vi "CSTK_Enum_Creator.vi"(10 "应用程序:菜单启动:VI":string, 11 "应用程序引用（本地）":refnum<vi>) -> ()   [LabVIEW 2015, in "CSTK_Enum Creator.lvlib"]
uses:
  CSTK_Enum Creator.lvlib
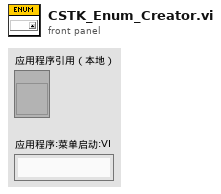
[diagram p1: front panel]
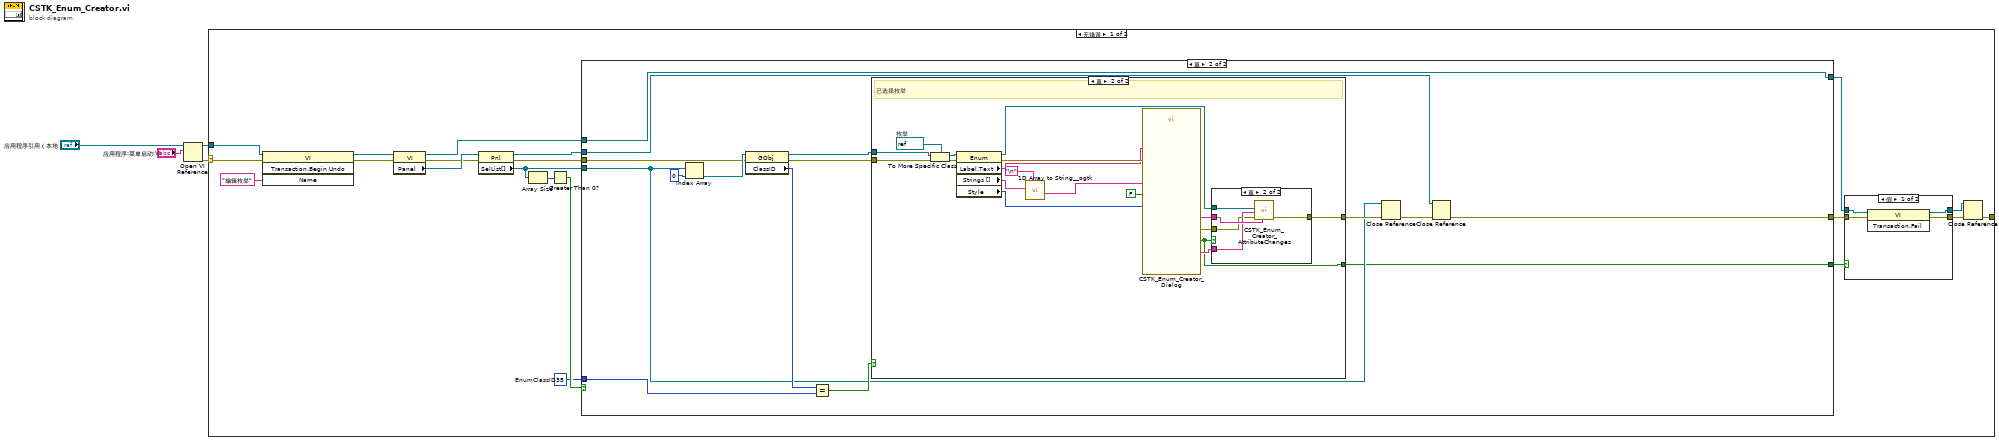
[diagram p0: block diagram]
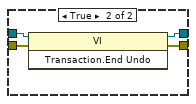
[diagram p2: hidden frame]
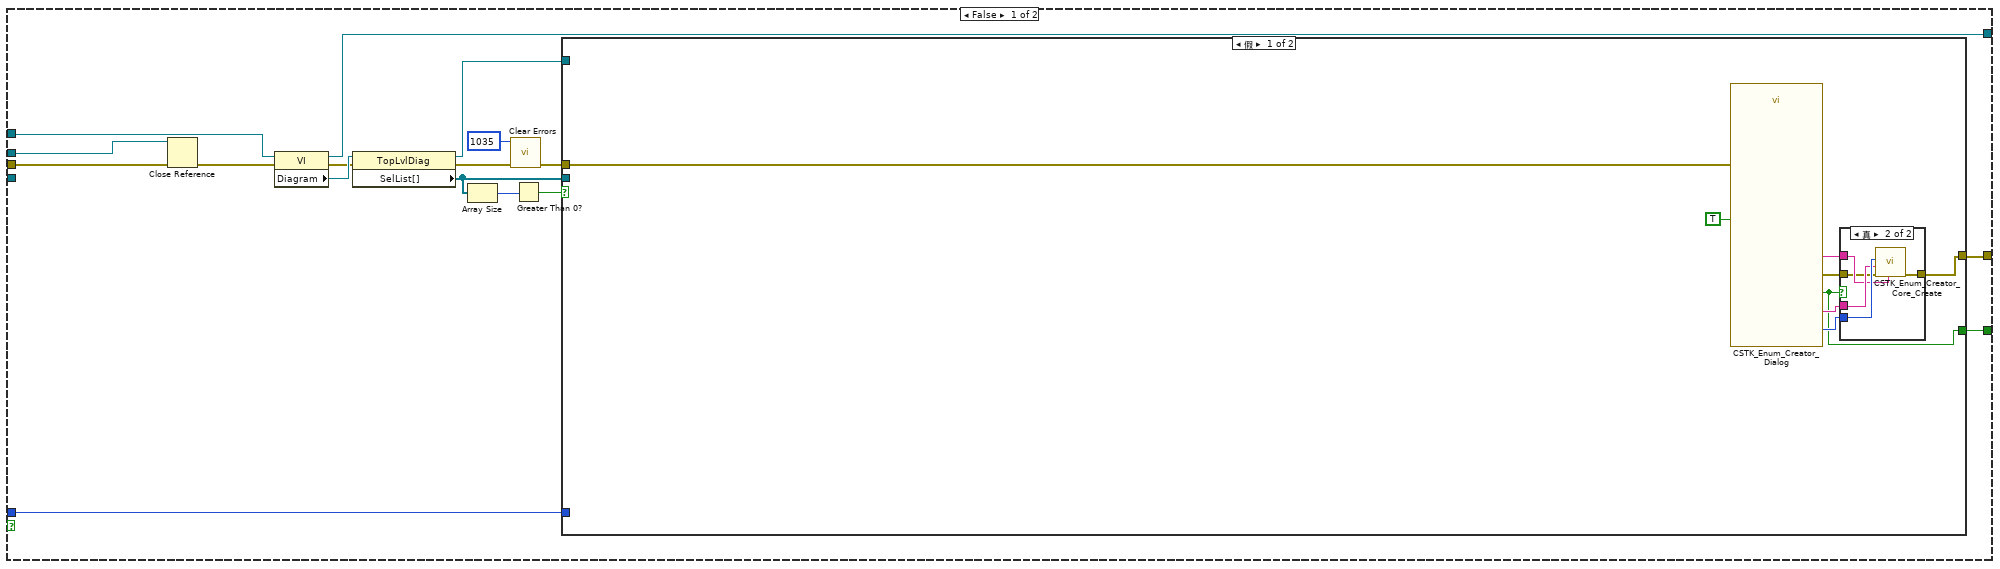
[diagram p3: hidden frame]
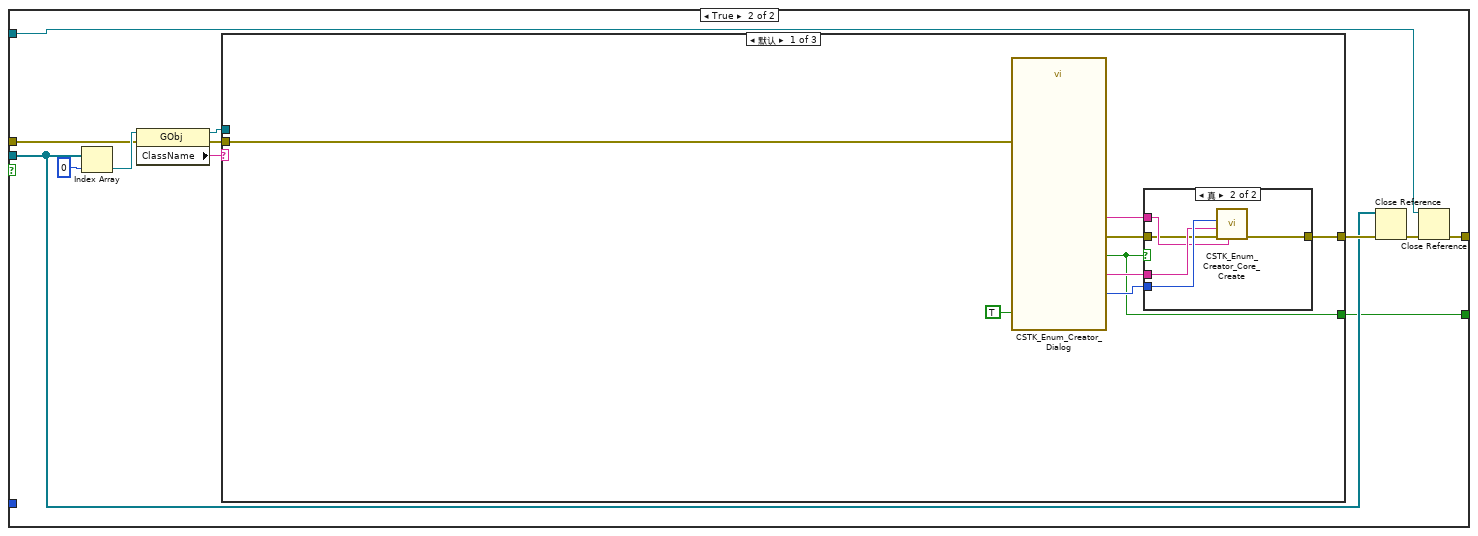
[diagram p5: hidden frame]
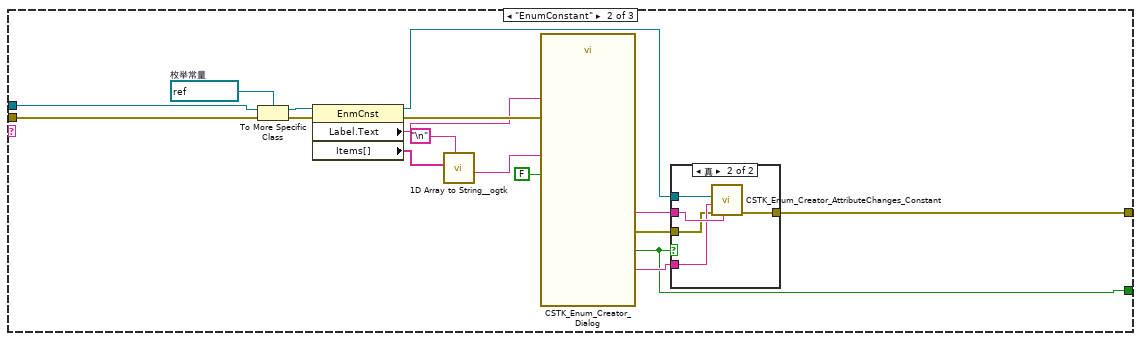
[diagram p7: hidden frame]
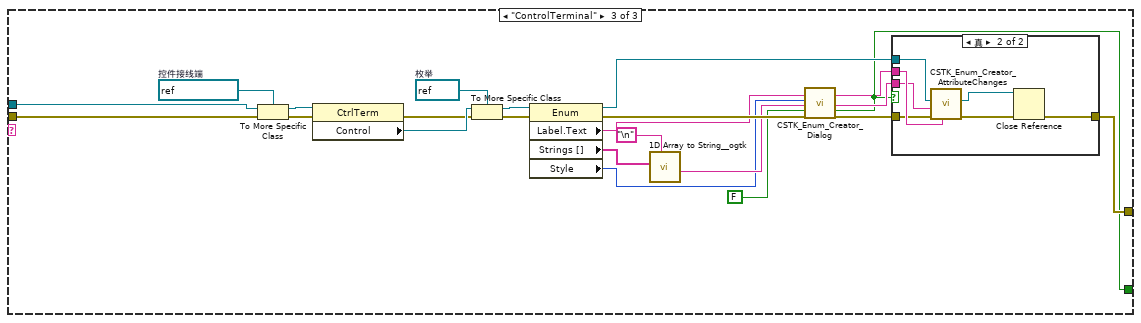
[diagram p9: hidden frame]
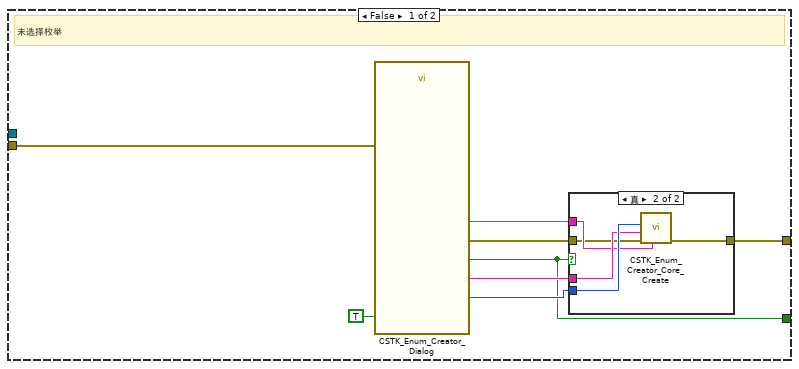
[diagram p11: hidden frame]
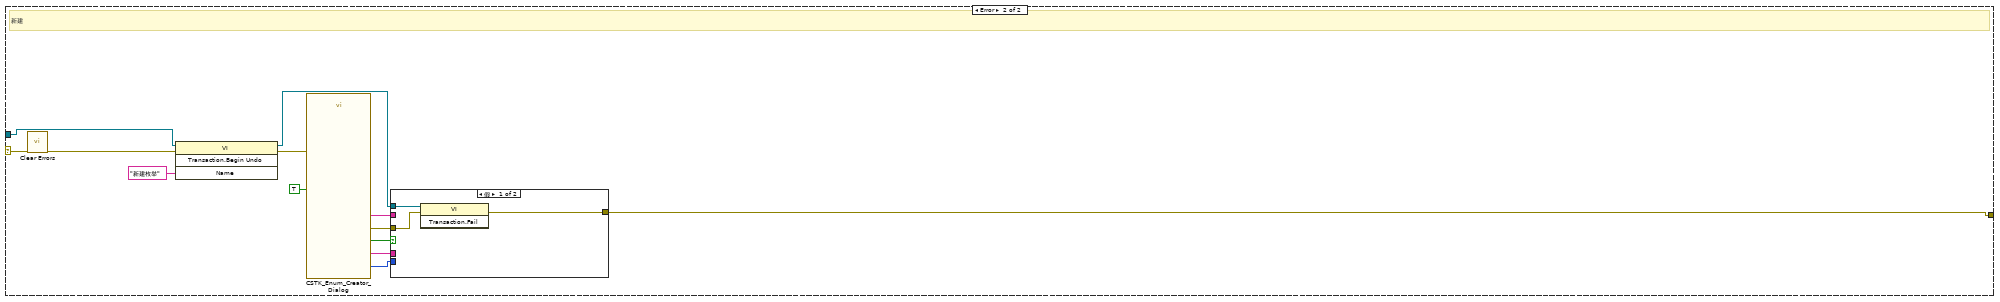
[diagram p14: hidden frame]
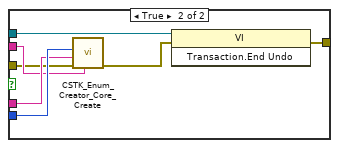
[diagram p15: hidden frame]
diagram:
  n1 = Open VI Reference(application reference (local)="应用程序引用（本地）", vi path="应用程序:菜单启动:VI") -> (vi reference=w1:refnum<vi>, error out=w3:errorcluster)  [unwired: 4 in]
  n2 = case shown="无错误" w3 {
    selector: w3 -> [w13 w209]
    tunnel: w1 -> [w14 w200]
    tunnel: [w21 w202] -> _
    frame No Error {
      w15 = u32 35  # EnumClassID
      n3 = invoke class="VI" method="Transaction.Begin Undo"(reference=w14, error in=w13, "Name"="编辑枚举" ("名称")) -> (reference out=w12:refnum<vi>, error out=w11:errorcluster)  [unwired: 1 in, 2 out]
      n4 = property class="VI"(reference=w12, error in=w11) -> (reference out=w17:refnum<vi>, error out=w22:errorcluster, "Panel"=w24:refnum<vi>)
      n5 = property class="Pnl"(reference=w24, error in=w22) -> (reference out=w16:refnum<vi>, error out=w23:errorcluster, "SelList[]"=w20:refnum<vi>[])
      n6 = Array Size(array=w20) -> (size(s)=w19:i32)
      n7 = Greater Than 0?(x=w19) -> (x > 0?=w18:bool)
      n8 = case shown="真" w18 {
        tunnel: w23 -> [w36 w153]
        tunnel: [w41 w147] -> w7
        tunnel: w20 -> [_ w150]
        tunnel: w17 -> [w49 w149]
        tunnel: [w46 w149] -> w9
        tunnel: w16 -> [w45 w146]
        tunnel: w15 -> [w38 w145]
        tunnel: [w35 w144] -> w5
        frame False {
          n9 = Close Reference(reference=w45, error in (no error)=w36) -> (error out=w44:errorcluster)
          n10 = property class="VI"(reference=w49, error in=w44) -> (reference out=w46:refnum<vi>, error out=w47:errorcluster, "Diagram"=w48:refnum<vi>)
          n11 = property class="TopLvlDiag"(reference=w48, error in=w47) -> (reference out=w37:refnum<vi>, error out=w40:errorcluster, "SelList[]"=w39:refnum<vi>[])
          n12 = Array Size(array=w39) -> (size(s)=w43:i32)
          n13 = call <vilib>:"Clear Errors.vi"("error in (no error)"=w40, "specific error code to clear (0: all)"=1035) -> ("error out"=w34:errorcluster)  [unwired: 4 in, 1 out]
          n14 = Greater Than 0?(x=w43) -> (x > 0?=w42:bool)
          n15 = case shown="假" w42 {
            tunnel: [w51 w73] -> w41
            tunnel: w34 -> [w52 w65]
            tunnel: w39 -> [_ w71]
            tunnel: w38 -> [_ _]
            tunnel: w37 -> [_ w70]
            tunnel: [w50 w64] -> w35
            frame False {
              n16 = call "CSTK_Enum_Creator_Dialog.vi"("新建？"=TRUE, "error in (no error)"=w52) -> ("标签名输出"=w54:string, "样式输出"=w56:u32, "项名输出"=w55:string, "确定"=w50:bool, "error out"=w53:errorcluster)  [unwired: 13 in]
              n17 = case shown="真" w50 {
                tunnel: w56 -> [_ w63]
                tunnel: w55 -> [_ w62]
                tunnel: w54 -> [_ w61]
                tunnel: w53 -> [w58 w60]
                tunnel: [w58 w59] -> w51
                frame False {
                }
                frame True {
                  n18 = call "CSTK_Enum_Creator_Core_Create.vi"("标签名"=w61, "错误输入（无错误）"=w60, "项名"=w62, "样式"=w63) -> ("错误输出"=w59:errorcluster)  [unwired: 7 in]
                }
              }
            }
            frame True {
              n19 = Index Array(array=w71, index=0 ("索引")) -> (element=w66:refnum<vi>)
              n20 = property class="GObj"(reference=w66, error in=w65) -> (reference out=w69:refnum<vi>, error out=w68:errorcluster, "ClassName"=w67:string)
              n21 = case shown="默认" w67 {
                tunnel: [w77 w94 w123] -> w72
                tunnel: w69 -> [_ w93 w118]
                tunnel: w68 -> [w78 w92 w117]
                tunnel: [w76 w90 w113] -> w64
                frame Default {
                  n22 = call "CSTK_Enum_Creator_Dialog.vi"("新建？"=TRUE, "error in (no error)"=w78) -> ("标签名输出"=w80:string, "样式输出"=w82:u32, "项名输出"=w81:string, "确定"=w76:bool, "error out"=w79:errorcluster)  [unwired: 13 in]
                  n23 = case shown="真" w76 {
                    tunnel: w82 -> [_ w89]
                    tunnel: w81 -> [_ w88]
                    tunnel: w80 -> [_ w87]
                    tunnel: w79 -> [w84 w86]
                    tunnel: [w84 w85] -> w77
                    frame False {
                    }
                    frame True {
                      n24 = call "CSTK_Enum_Creator_Core_Create.vi"("标签名"=w87, "错误输入（无错误）"=w86, "项名"=w88, "样式"=w89) -> ("错误输出"=w85:errorcluster)  [unwired: 7 in]
                    }
                  }
                }
                frame "EnumConstant" {
                  w91 = refnum<vi> refnum  # 枚举常量
                  n25 = To More Specific Class(target class=w91, reference=w93, error in=w92) -> (specific class reference=w106:refnum<vi>, error out=w105:errorcluster)
                  n26 = property class="EnmCnst"(reference=w106, error in=w105) -> (reference out=w99:refnum<vi>, error out=w104:errorcluster, "Label.Text"=w103:string, "Items[]"=w102:string[])
                  n27 = call <userlib>:"1D Array to String__ogtk.vi"("delimiter (Tab)"="\n", "Array of Strings"=w102) -> ("delimited string"=w100:string)  [unwired: 9 in]
                  n28 = call "CSTK_Enum_Creator_Dialog.vi"("标签名输入"=w103, "项名输入"=w100, "新建？"=FALSE, "error in (no error)"=w104) -> ("标签名输出"=w98:string, "项名输出"=w97:string, "确定"=w90:bool, "error out"=w96:errorcluster)  [unwired: 11 in, 1 out]
                  n29 = case shown="真" w90 {
                    tunnel: w99 -> [_ w112]
                    tunnel: w98 -> [_ w111]
                    tunnel: w97 -> [_ w110]
                    tunnel: w96 -> [w107 w109]
                    tunnel: [w107 w108] -> w94
                    frame False {
                    }
                    frame True {
                      n30 = call "CSTK_Enum_Creator_AttributeChanges_Constant.vi"("标签名"=w111, "错误输入（无错误）"=w109, "项名"=w110, "EnumCnst输入"=w112) -> ("错误输出"=w108:errorcluster)  [unwired: 5 in, 2 out]
                    }
                  }
                }
                frame "ControlTerminal" {
                  w120 = refnum<vi> refnum  # 控件接线端
                  w122 = refnum<vi> refnum  # 枚举
                  n31 = To More Specific Class(target class=w120, reference=w118, error in=w117) -> (specific class reference=w119:refnum<vi>, error out=w116:errorcluster)
                  n32 = property class="CtrlTerm"(reference=w119, error in=w116) -> (error out=w114:errorcluster, "Control"=w115:refnum<vi>)  [unwired: 1 out]
                  n33 = To More Specific Class(target class=w122, reference=w115, error in=w114) -> (specific class reference=w135:refnum<vi>, error out=w134:errorcluster)
                  n34 = property class="Enum"(reference=w135, error in=w134) -> (reference out=w128:refnum<vi>, error out=w133:errorcluster, "Label.Text"=w132:string, "Strings []"=w131:string[], "Style"=w121:u32)
                  n35 = call <userlib>:"1D Array to String__ogtk.vi"("delimiter (Tab)"="\n", "Array of Strings"=w131) -> ("delimited string"=w129:string)  [unwired: 9 in]
                  n36 = call "CSTK_Enum_Creator_Dialog.vi"("标签名输入"=w132, "样式输入"=w121, "项名输入"=w129, "新建？"=FALSE, "error in (no error)"=w133) -> ("标签名输出"=w127:string, "项名输出"=w126:string, "确定"=w113:bool, "error out"=w125:errorcluster)  [unwired: 10 in, 1 out]
                  n37 = case shown="真" w113 {
                    tunnel: w128 -> [_ w143]
                    tunnel: w127 -> [_ w142]
                    tunnel: w126 -> [_ w141]
                    tunnel: w125 -> [w136 w140]
                    tunnel: [w136 w138] -> w123
                    frame False {
                    }
                    frame True {
                      n38 = call "CSTK_Enum_Creator_AttributeChanges.vi"("标签名"=w142, "错误输入（无错误）"=w140, "项名"=w141, "Enum输入"=w143) -> ("错误输出"=w139:errorcluster, "Enum输出"=w137:refnum<vi>)  [unwired: 5 in, 1 out]
                      n39 = Close Reference(reference=w137, error in (no error)=w139) -> (error out=w138:errorcluster)
                    }
                  }
                }
              }
              n40 = Close Reference(reference=w71, error in (no error)=w72) -> (error out=w74:errorcluster)
              n41 = Close Reference(reference=w70, error in (no error)=w74) -> (error out=w73:errorcluster)
            }
          }
        }
        frame True {
          n42 = Index Array(array=w150, index=0 ("索引")) -> (element=w157:refnum<vi>)
          n43 = property class="GObj"(reference=w157, error in=w153) -> (reference out=w155:refnum<vi>, error out=w154:errorcluster, "ClassID"=w151:u32)
          n44 = Equal?(x=w151, y=w145) -> (x = y?=w156:bool)
          n45 = case shown="真" w156 {
            tunnel: w155 -> [_ w190]
            tunnel: w154 -> [w160 w188]
            tunnel: [w161 w174] -> w152
            tunnel: [w159 w173] -> w144
            frame False {
              # "未选择枚举"
              n46 = call "CSTK_Enum_Creator_Dialog.vi"("新建？"=TRUE, "error in (no error)"=w160) -> ("标签名输出"=w163:string, "样式输出"=w165:u32, "项名输出"=w164:string, "确定"=w159:bool, "error out"=w162:errorcluster)  [unwired: 13 in]
              n47 = case shown="真" w159 {
                tunnel: w165 -> [_ w172]
                tunnel: w164 -> [_ w171]
                tunnel: w163 -> [_ w170]
                tunnel: w162 -> [w167 w169]
                tunnel: [w167 w168] -> w161
                frame False {
                }
                frame True {
                  n48 = call "CSTK_Enum_Creator_Core_Create.vi"("标签名"=w170, "错误输入（无错误）"=w169, "项名"=w171, "样式"=w172) -> ("错误输出"=w168:errorcluster)  [unwired: 7 in]
                }
              }
            }
            frame True {
              w189 = refnum<vi> refnum  # 枚举
              # "已选择枚举"
              n49 = To More Specific Class(target class=w189, reference=w190, error in=w188) -> (specific class reference=w187:refnum<vi>, error out=w186:errorcluster)
              n50 = property class="Enum"(reference=w187, error in=w186) -> (reference out=w179:refnum<vi>, error out=w185:errorcluster, "Label.Text"=w183:string, "Strings []"=w182:string[], "Style"=w184:u32)
              n51 = call <userlib>:"1D Array to String__ogtk.vi"("delimiter (Tab)"="\n", "Array of Strings"=w182) -> ("delimited string"=w180:string)  [unwired: 9 in]
              n52 = call "CSTK_Enum_Creator_Dialog.vi"("标签名输入"=w183, "样式输入"=w184, "项名输入"=w180, "新建？"=FALSE, "error in (no error)"=w185) -> ("标签名输出"=w178:string, "项名输出"=w177:string, "确定"=w173:bool, "error out"=w176:errorcluster)  [unwired: 10 in, 1 out]
              n53 = case shown="真" w173 {
                tunnel: w179 -> [_ w196]
                tunnel: w178 -> [_ w195]
                tunnel: w177 -> [_ w194]
                tunnel: w176 -> [w191 w193]
                tunnel: [w191 w192] -> w174
                frame False {
                }
                frame True {
                  n54 = call "CSTK_Enum_Creator_AttributeChanges.vi"("标签名"=w195, "错误输入（无错误）"=w193, "项名"=w194, "Enum输入"=w196) -> ("错误输出"=w192:errorcluster)  [unwired: 5 in, 2 out]
                }
              }
            }
          }
          n55 = Close Reference(reference=w150, error in (no error)=w152) -> (error out=w148:errorcluster)
          n56 = Close Reference(reference=w146, error in (no error)=w148) -> (error out=w147:errorcluster)
        }
      }
      n57 = case shown="假" w5 {
        tunnel: w7 -> [w27 w30]
        tunnel: [w26 w31] -> w6
        tunnel: w9 -> [w28 w32]
        tunnel: [w25 w29] -> w8
        frame False {
          n58 = invoke class="VI" method="Transaction.Fail"(reference=w28, error in=w27) -> (reference out=w25:refnum<vi>, error out=w26:errorcluster)  [unwired: 1 in, 1 out]
        }
        frame True {
          n59 = invoke class="VI" method="Transaction.End Undo"(reference=w32, error in=w30) -> (reference out=w29:refnum<vi>, error out=w31:errorcluster)  [unwired: 1 in, 1 out]
        }
      }
      n60 = Close Reference(reference=w8, error in (no error)=w6) -> (error out=w21:errorcluster)
    }
    frame Error {
      # "新建"
      n61 = call <vilib>:"Clear Errors.vi"("error in (no error)"=w209) -> ("error out"=w201:errorcluster)  [unwired: 5 in, 1 out]
      n62 = invoke class="VI" method="Transaction.Begin Undo"(reference=w200, error in=w201, "Name"="新建枚举" ("名称")) -> (reference out=w197:refnum<vi>, error out=w199:errorcluster)  [unwired: 1 in, 2 out]
      n63 = call "CSTK_Enum_Creator_Dialog.vi"("新建？"=TRUE, "error in (no error)"=w199) -> ("标签名输出"=w205:string, "样式输出"=w207:u32, "项名输出"=w206:string, "确定"=w203:bool, "error out"=w204:errorcluster)  [unwired: 13 in]
      n64 = case shown="假" w203 {
        tunnel: w207 -> [_ w219]
        tunnel: w206 -> [_ w218]
        tunnel: w205 -> [_ w217]
        tunnel: w204 -> [w211 w216]
        tunnel: [w210 w213] -> w202
        tunnel: w197 -> [w212 w214]
        frame False {
          n65 = invoke class="VI" method="Transaction.Fail"(reference=w212, error in=w211) -> (error out=w210:errorcluster)  [unwired: 1 in, 2 out]
        }
        frame True {
          n66 = call "CSTK_Enum_Creator_Core_Create.vi"("标签名"=w217, "错误输入（无错误）"=w216, "项名"=w218, "样式"=w219) -> ("错误输出"=w215:errorcluster)  [unwired: 7 in]
          n67 = invoke class="VI" method="Transaction.End Undo"(reference=w214, error in=w215) -> (error out=w213:errorcluster)  [unwired: 1 in, 2 out]
        }
      }
    }
  }
